vi "MGCC_BlkStart_Output_Flag.vi"(9 "BKS_falilure":bool) -> (1 "Boolean 3":bool)   [LabVIEW 2016]
doc: "-----------------------------------------------------------------------------------------------------------------------\nCopyright <2019> <The University of Tennessee at Knoxville and the University of Tennessee Research Foundation>\nThis software is released under BSD-3 \nhttps://opensource.org/licenses/BSD-3-Clause \nAdditional license options available at https://utrf.tennessee.edu/industry/sample-agreements/\n-----------------------------------------------------------------------------------------------------------------------"
panel:
  out "Boolean":bool
  out "Boolean 2":bool
  in  "i>=20?":bool
  in  "=1?":bool
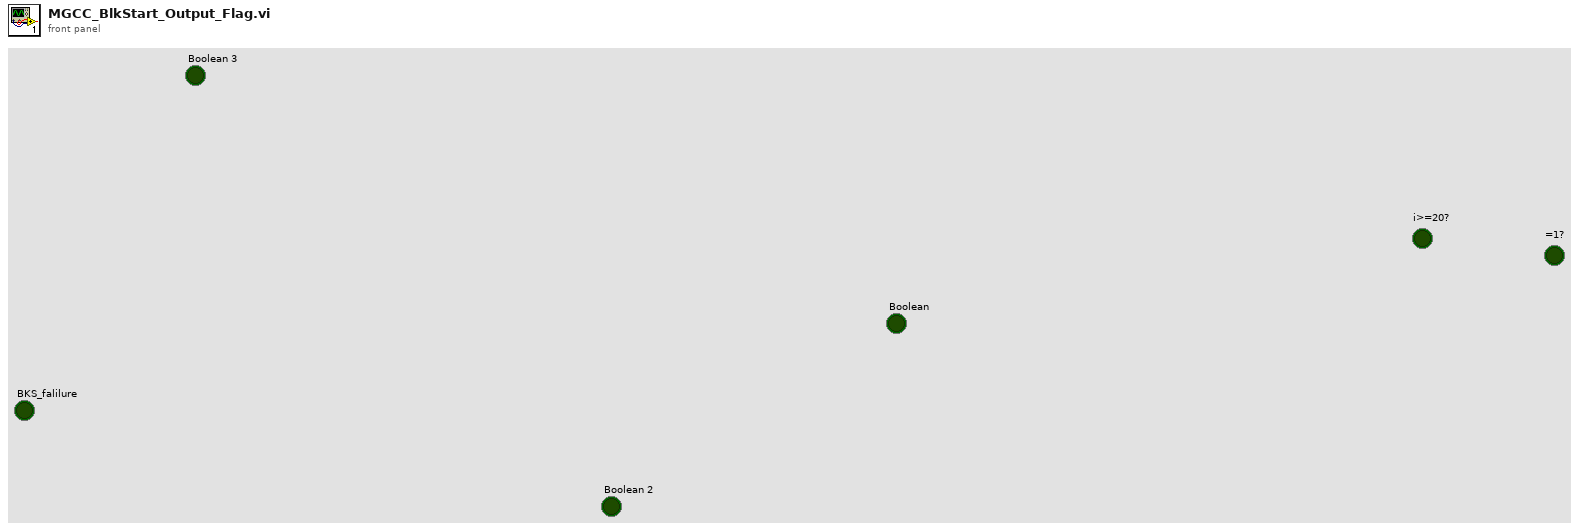
[diagram p1: front panel]
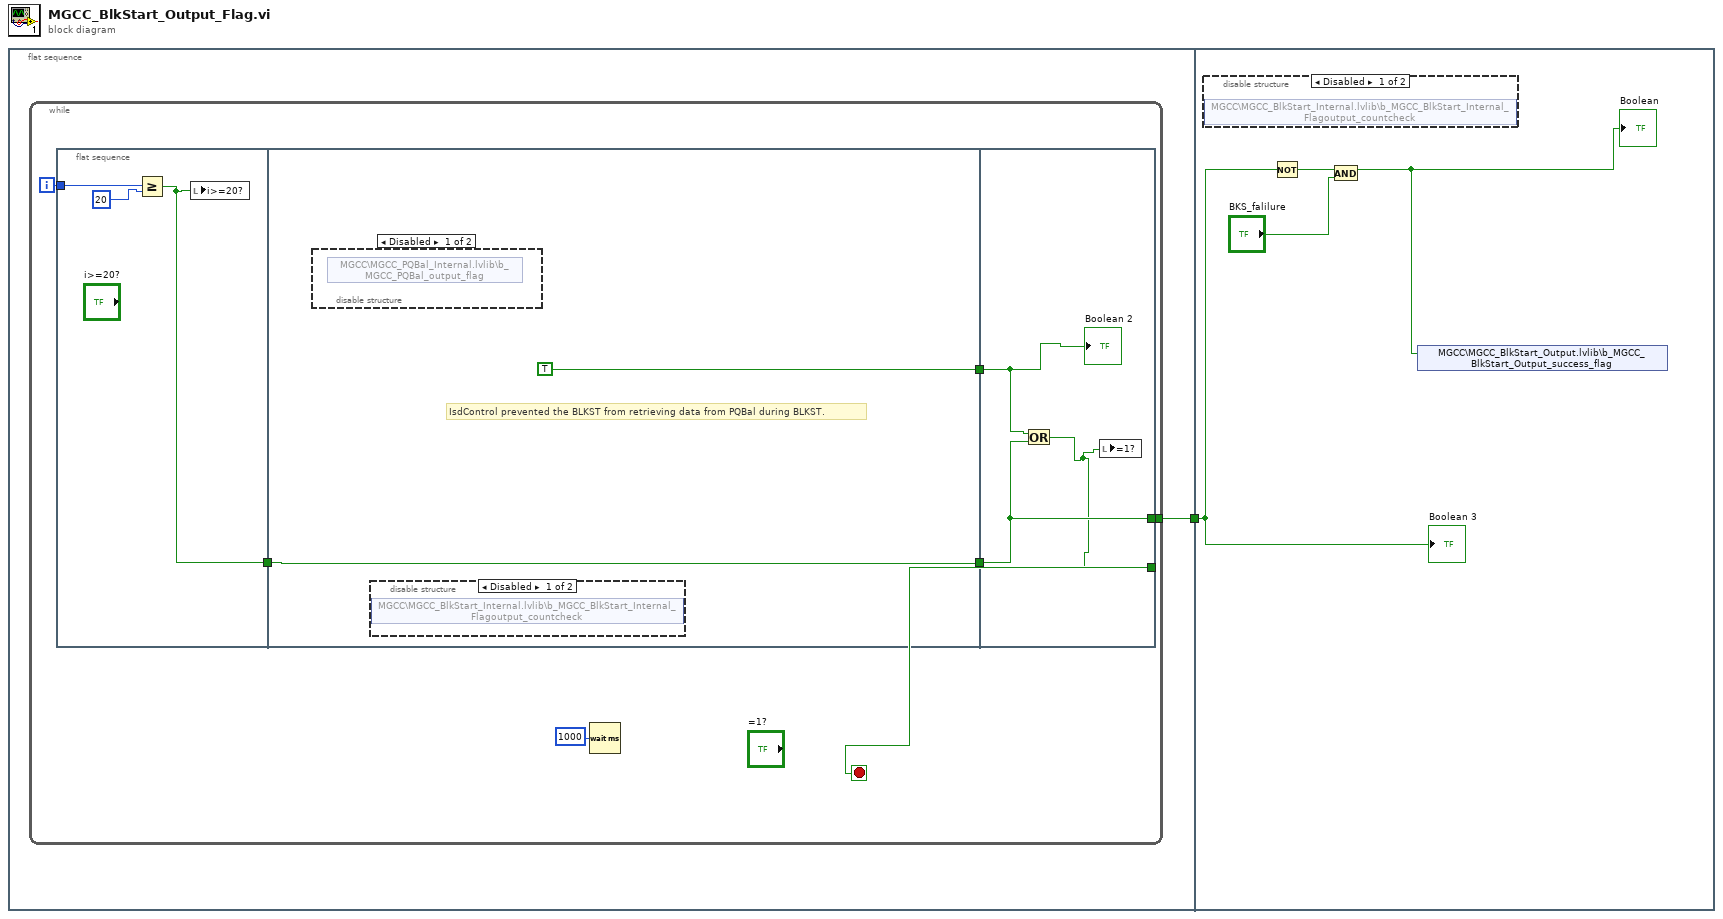
[diagram p0: block diagram]
diagram:
  n1 = flat-sequence {
    tunnel: [w2] -> w1
    tunnel: w1 -> [w20]
    frame #0 {
      n2 = while {
        tunnel: [w5] -> w2
        i -> [w8]
        stop <- w3 stop-if-true
        n3 = flat-sequence {
          tunnel: w8 -> [w12]
          tunnel: [w10] -> w4
          tunnel: [w14] -> w7
          tunnel: [TRUE ("Boolean")] -> w6
          tunnel: w4 -> [w14]
          tunnel: w7 -> [w16]
          tunnel: w6 -> [w17]
          tunnel: [w16] -> w5
          tunnel: [w15] -> w3
          frame #0 {
            n4 = Greater Or Equal?(x=w12, y=20) -> (x >= y?=w10:bool)
            n5 = local write "i>=20?"(w10) -> ()
          }
          frame #1 {
            # "IsdControl prevented the BLKST from retrieving data from PQBal during BLKST."
            n6 = disable-structure shown="Disabled" {
              frame Disabled {
                n7 = shared-variable "MGCC\\MGCC_PQBal_Internal.lvlib\\b_MGCC_PQBal_output_flag"() -> ()  [unwired: 1 in, 2 out]
              }
              frame Enabled {
              }
            }
            n8 = disable-structure shown="Disabled" {
              frame Disabled {
                n9 = shared-variable "MGCC\\MGCC_BlkStart_Internal.lvlib\\b_MGCC_BlkStart_Internal_Flagoutput_countcheck"() -> ()  [unwired: 2 in, 1 out]
              }
              frame Enabled {
              }
            }
          }
          frame #2 {
            n10 = Or(x=w17, y=w16) -> (x .or. y?=w15:bool)
            n11 = local write "=1?"(w15) -> ()
            "Boolean 2" <- w17
          }
        }
        n12 = Wait (ms)(milliseconds to wait=1000) -> ()  [unwired: 1 out]
      }
    }
    frame #1 {
      n13 = disable-structure shown="Disabled" {
        frame Disabled {
          n14 = shared-variable "MGCC\\MGCC_BlkStart_Internal.lvlib\\b_MGCC_BlkStart_Internal_Flagoutput_countcheck"() -> ()  [unwired: 1 in, 2 out]
        }
        frame Enabled {
        }
      }
      n15 = Not(x=w20) -> (.not. x?=w21:bool)
      n16 = And(x=w21, y="BKS_falilure") -> (x .and. y?=w19:bool)
      "Boolean" <- w19
      n17 = shared-variable "MGCC\\MGCC_BlkStart_Output.lvlib\\b_MGCC_BlkStart_Output_success_flag"(w19) -> ()  [unwired: 1 in, 1 out]
      "Boolean 3" <- w20
    }
  }
